vi "HTVacuum.ReadVariables.vi"(0 "i ref in":refnum<vi>, 5 "error in (no error)":errorcluster) -> (14 "i ref out":refnum<vi>, 16 "U-VAR values":i32[](array[numeric]), 19 "error out":errorcluster)   [LabVIEW 2014, in "HTVacuum.lvlib"]
doc: "Reads the attribute data of the object after the access to the data has been locked by the \"acquire\" method. If the attribute data has been locked already, this methods waits until the attribute data is unlocked or there is a timeout.\n\nThe attribute data must be unlocked using the methods \"release\" or \"set modified data\".\n\nLicense Agreement for this software:\n\nCopyright (C)\nGesellschaft für Schwerionenforschung, GSI\nPlanckstr. 1\n64291 Darmstadt\nGermany\n\nContact: D.Beck@gsi.de \n\nThis program is free software; you can redistribute it and/or modify it under the terms of the GNU General Public License as published by the Free Software Foundation; either version 2 of the license, or (at your option) any later version.\n\nThis program is distributed in the hope that it will be useful, but WITHOUT ANY WARRANTY; without even the implied warranty of MERCHANTABILITY or FITNESS FOR A PARTICULAR PURPOSE. See the GNU General License for more details (http://www.gnu.org).\n\nGesellschaft für Schwerionenforschung, GSI\nPlanckstr. 1, 64291 Darmstadt, Germany\nFor all questions and ideas contact: M.Richter@gsi.de, H.Brand@gsi.de or D.Beck@gsi.de.\nLast update: 17-JUN-2004"
uses:
  HTVacuum.lvlib
  instr.lib/M&M/_ica01/ica-Lib SubVIs/M&M SubVIs/M&M USB Var Read U-Variables.vi
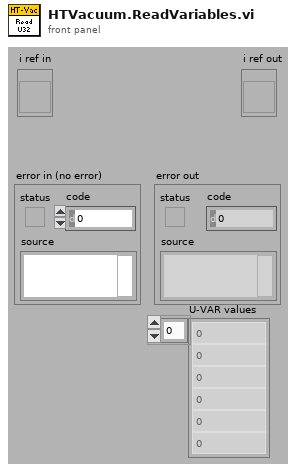
[diagram p1: front panel]
types:
  T1 = typedef "HTVacuum.lvlib/HTVacuum.i attribute.ctl" = cluster{"USB-Handle":cluster{"Write handle":i32, "Read handle":i32}}
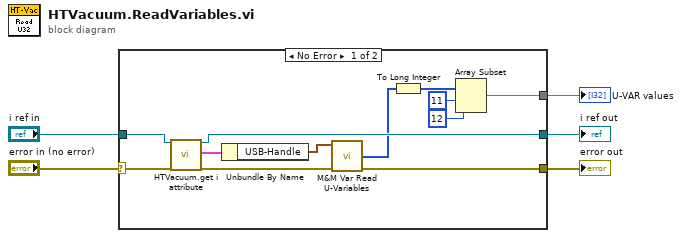
[diagram p0: block diagram]
diagram:
  n1 = case shown="No Error" "error in (no error)" {
    selector: "error in (no error)" -> [w16 w19]
    tunnel: [w17 w19] -> w4
    tunnel: "i ref in" -> [w14 w18]
    tunnel: [w13 w18] -> w2
    tunnel: [w10 _] -> w1
    frame No Error {
      n2 = call "HTVacuum.get i attribute.vi"("i ref in"=w14, "error in (no error)"=w16) -> ("i ref out"=w13:refnum<vi>, "i attribute"=w12:T1, "error out"=w15:errorcluster)  [unwired: 15 in]
      n3 = Unbundle By Name(w12) -> ("USB-Handle"=w11:cluster{"Write handle":i32, "Read handle":i32})
      n4 = call-poly "M&M Var Read U-Variables.vi"("error in (no error)"=w15, "USB-Handles in"=w11) -> ("error out"=w17:errorcluster, "U-VAR values"=w8:u32[])  [unwired: 6 in, 1 out]
      n5 = To Long Integer(number=w8) -> (32bit integer=w7:i32[])
      n6 = Array Subset(array=w7, index=11 ("length"), length=12) -> (w10:i32[])
    }
    frame Error {
    }
  }
  "error out" <- w4
  "i ref out" <- w2
  "U-VAR values" <- w1
